vi "Validate Device ID Code1.vi"(10 "read device ID code":T1(ring), 11 "deivce conformity level":u8(ring)=1 items=["None"=0, "Basic Stream"=1, "Regular Stream"=2, "Extended Stream"=3, "Basic Stream/Individual"=129, "Regular Stream/Individual"=130, "Extended Stream/Individual"=131]) -> (3 "valid?":bool)   [LabVIEW 2021, in "NI_modbus_upd.lvlib" / "Standard Data Model1.lvclass"]
doc: "This confirms that the device can accept the read device id request type."
uses:
  Standard Data Model1.lvclass
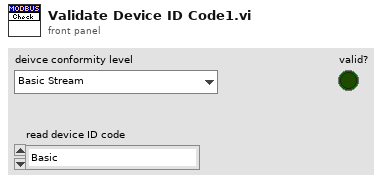
[diagram p1: front panel]
types:
  T1 = enum8{"Basic", "Regular", "Extended", "Specific"}
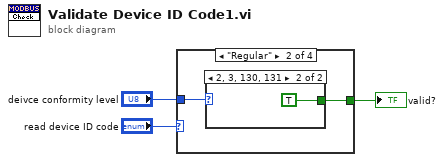
[diagram p0: block diagram]
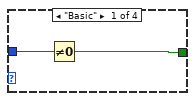
[diagram p2: hidden frame]
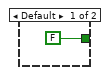
[diagram p3: hidden frame]
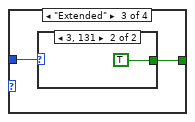
[diagram p4: hidden frame]
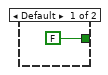
[diagram p5: hidden frame]
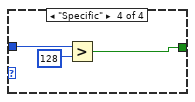
[diagram p6: hidden frame]
diagram:
  n1 = case shown="\"Regular\"" "read device ID code" {
    tunnel: "deivce conformity level" -> [w5 w7 w11 w16]
    tunnel: [w4 w6 w10 w14] -> w1
    frame "Basic" {
      n2 = Not Equal To 0?(x=w5) -> (x != 0?=w4:bool)
    }
    frame "Regular" {
      n3 = case shown="2, 3, 130, 131" w7 {
        tunnel: [FALSE TRUE] -> w6
        frame Default {
        }
        frame 2, 3, 130, 131 {
        }
      }
    }
    frame "Extended" {
      n4 = case shown="3, 131" w11 {
        tunnel: [FALSE TRUE] -> w10
        frame Default {
        }
        frame 3, 131 {
        }
      }
    }
    frame "Specific" {
      n5 = Greater?(x=w16, y=u8 128) -> (0:w14:bool)
    }
  }
  "valid?" <- w1
